vi "Get VI Icon.vi"(8 "error in (no error)":errorcluster, 11 "VI Refnum in":refnum<vi>) -> (0 "error out":errorcluster, 2 "Icon":refnum<class "Icon.lvclass">, 3 "VI Refnum out":refnum<vi>)   [LabVIEW 2020, in "LabVIEW Icon API.lvlib"]
doc: "Returns the LabVIEW Icon class of the VI.\nIf the VI doesn't have any stored data, the default LabVIEW Icon class is returned instead."
uses:
  LabVIEW Icon API.lvlib
  lv_icon/Classes/Icon/Icon.lvclass
  lv_icon/Controls/Alignment.ctl
  lv_icon/Controls/Font.ctl
  lv_icon/Controls/BodyText.ctl
  lv_icon/lv_icon.lvlib
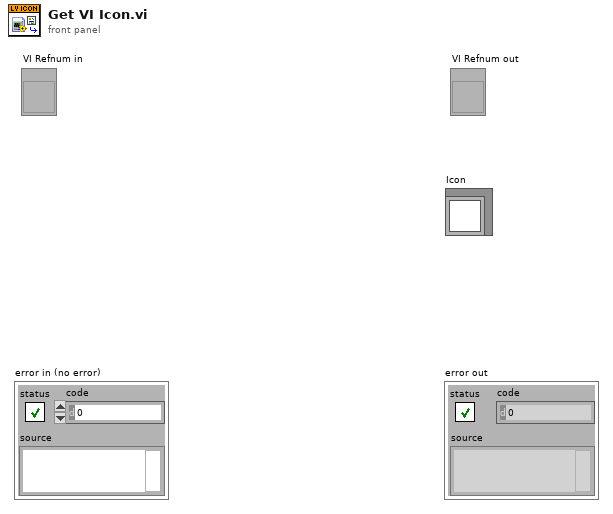
[diagram p1: front panel]
types:
  T1 = typedef "BodyText.ctl" = cluster{"Line 1 text":string, "Line 2 text":string, "Line 3 text":string, "Line 4 text":string, "Line 1 color":u32, "Line 2 color":u32, "Line 3 color":u32, "Line 4 color":u32, "Body Text Spec":cluster{"Font":T2, "Alignment":T3, "Size":u8}, "Center text vertically":bool, "Capitalize Text":bool}
  T2 = typedef "Font.ctl" = string
  T3 = typedef "Alignment.ctl" = u16
  T4 = typedef "LabVIEW Icon Stored Information.ctl" = cluster{"Text Visible?":bool, "Text Opacity":u8, "Templ Visible?":bool, "Templ Opacity":u8, "Relative Path from 1 to 2":path, "Image":picture, "All User Layers":refnum<class "Layer.lvclass">[], "Body Text":T1}
  T5 = typedef "imagedata.ctl" = cluster{"image type":i32, "image depth":i32, "image":u8[], "mask":u8[], "colors":u32[], "Rectangle":cluster{"left":i16, "top":i16, "right":i16, "bottom":i16}}
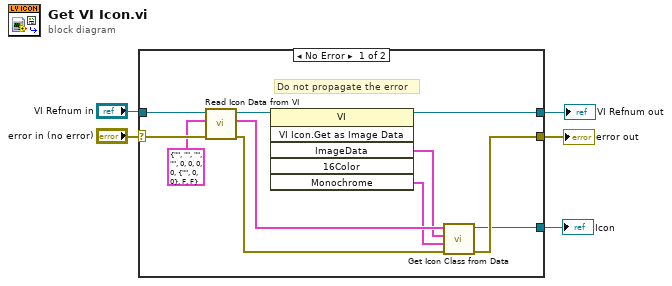
[diagram p0: block diagram]
diagram:
  n1 = case shown="No Error" "error in (no error)" {
    selector: "error in (no error)" -> [w16 w17]
    tunnel: [w12 w17] -> w2
    tunnel: "VI Refnum in" -> [w15 w18]
    tunnel: [w8 w18] -> w3
    tunnel: [w11 _] -> w1
    frame No Error {
      # "Do not propagate the error"
      n2 = call "Read Icon Data from VI.vi"("error in (no error)"=w16, "Default body text"=T1 {"Line 1 text"="", "Line 2 text"="", "Line 3 text"="", "Line 4 text"="", "Line 1 color"=0, "Line 2 color"=0, "Line 3 color"=0, "Line 4 color"=0, "Body Text Spec"={"Font"="", "Alignment"=0, "Size"=0}, "Center text vertically"=FALSE, "Capitalize Text"=FALSE}, "VI Ref in"=w15) -> ("error out"=w13:errorcluster, "Data"=w9:T4, "VI Ref out"=w10:refnum<vi>)  [unwired: 6 in]
      n3 = invoke class="VI" method="VI Icon.Get as Image Data"(reference=w10) -> (reference out=w8:refnum<vi>, "ImageData"=w7:T5, "Monochrome"=w6:T5)  [unwired: 5 in, 3 out]
      n4 = call "Get Icon Class from Data.vi"("error in (no error)"=w13, "BW Icon"=w6, "Color Icon"=w7, "Icon Data"=w9) -> ("error out"=w12:errorcluster, "Icon out"=w11:refnum<class "Icon.lvclass">)  [unwired: 6 in]
    }
    frame Error {
    }
  }
  "error out" <- w2
  "Icon" <- w1
  "VI Refnum out" <- w3
